vi "e.gate HighSpeedPort Diagnostics Full.vi"(0 "e.gate Configuration":T1 {"StartTime" format="%#.10f"; "dActTimeToSecondFactor" format="%#.10f"; "StartTimeToDayFactor" format="%#_10f"}, 11 "error in (no error)":errorcluster) -> (4 "e.gate Configuration out":T1 {"StartTime" format="%#.10f"; "dActTimeToSecondFactor" format="%#.10f"; "StartTimeToDayFactor" format="%#_10f"}, 6 "e.gate Interface Diagnostic Data":T9={"Interface Kind"=["Fieldbus", "Internal System", "Internal System", "ExternalUART", "ExternalUART", "ExternalUART"], "Interface Index"=[0, 0, 0, 0, 1, 2], "Cycles Count"=[280401, 280401, 280401, 280401, 14024, 280401], "Error Count"=[0, 0, 0, 0, 0, 0], "DeltaTimeS"=[1402.004973, 1402.004982, 1402.004982, 1402.004982, 1402.004983, 1402.004983]}, 8 "e.gate Transport Diagnostic Data":T8, 10 "e.gate Variable Diagnostic Data":T7, 15 "error out":errorcluster)   [LabVIEW 2016]
uses:
  e.gate Diagnostic Interface Data.ctl
  e.gate Diagnostic Transport Data.ctl
  e.gate Diagnostic Variable Data.ctl
  e.gate Configuration.ctl
  e.gate Channel Data.ctl
  e.gate Data Type.ctl
  e.gate Protocol Type.ctl
  e.gate Module  Data.ctl
  e.gateHSP_DLLhandle.ctl
panel:
  out "Remaining Data":u8[](array[numeric])
  out "Structure ID":i8
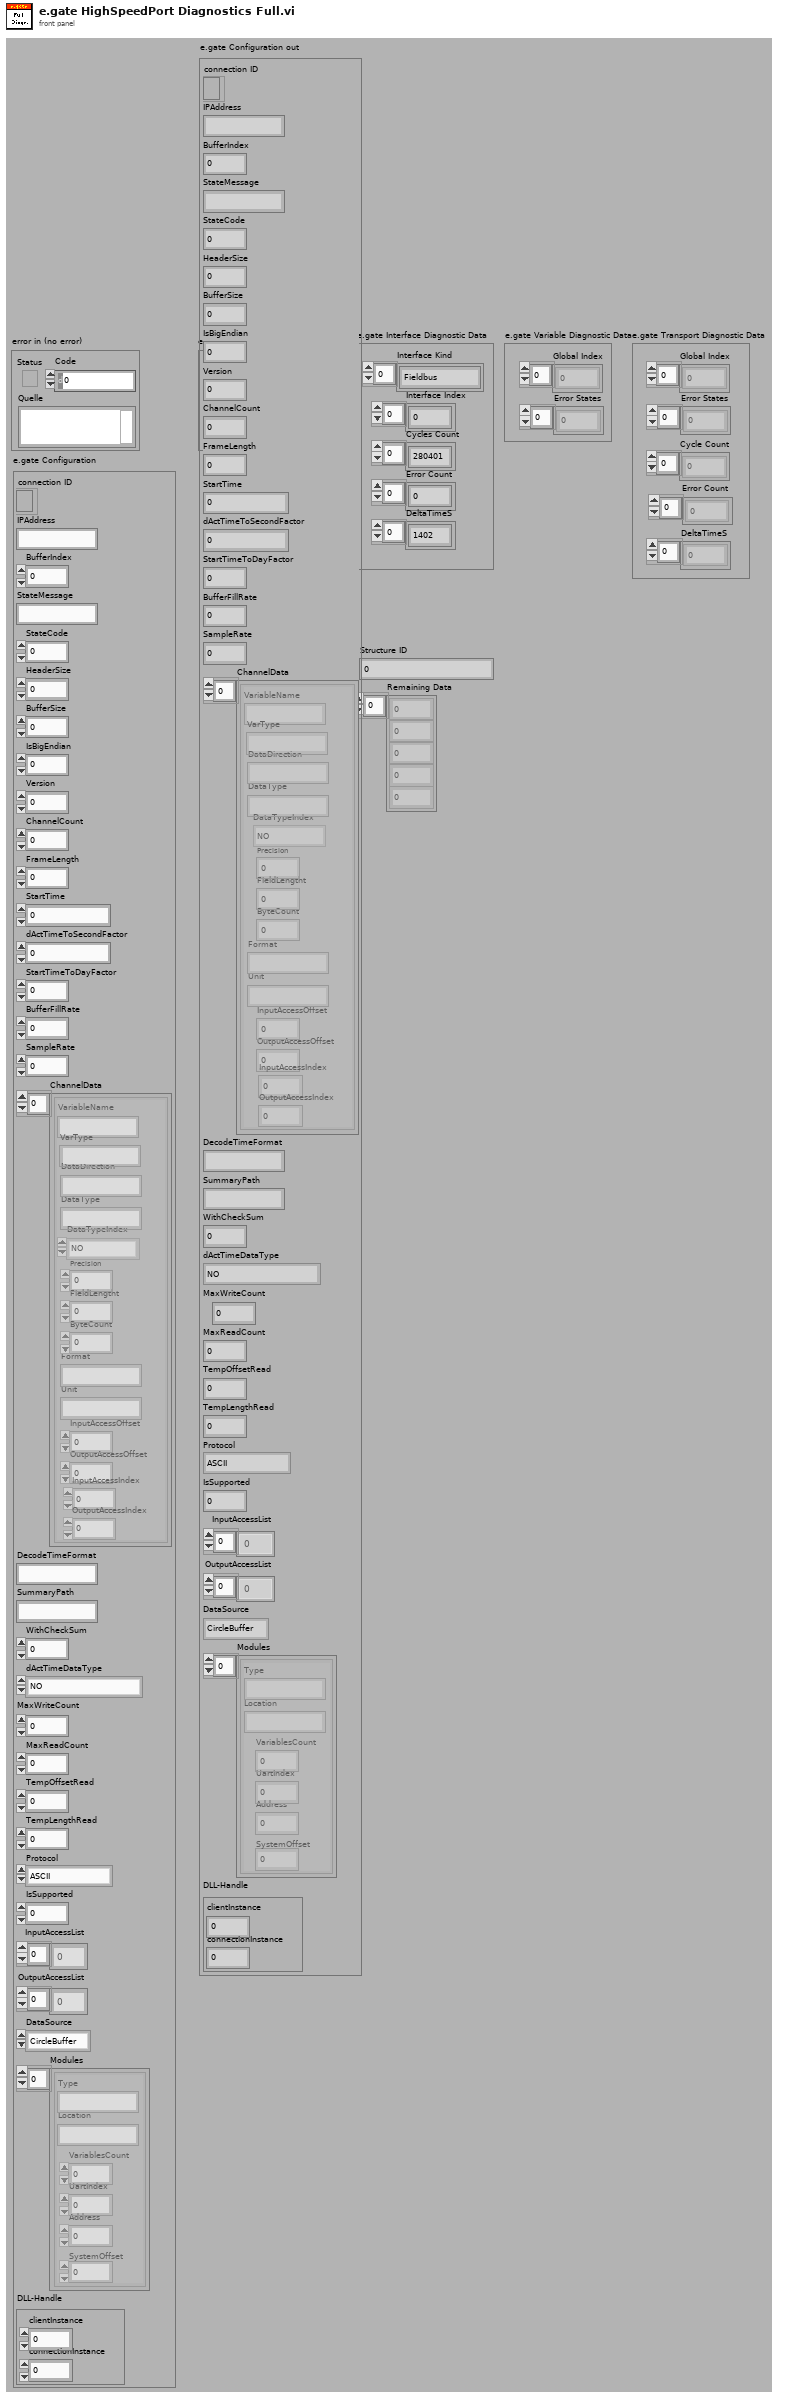
[diagram p1: front panel]
types:
  T1 = typedef "e.gate Configuration.ctl" = cluster{"connection ID":refnum<k5>, "IPAddress":string, "BufferIndex":i32, "StateMessage":string, "StateCode":i8, "HeaderSize":i32, "BufferSize":i32, "IsBigEndian":i32, "Version":i32, "ChannelCount":i32, "FrameLength":i32, "StartTime":dbl, "dActTimeToSecondFactor":dbl, "StartTimeToDayFactor":dbl, "BufferFillRate":dbl, "SampleRate":dbl, "ChannelData":T2[], "DecodeTimeFormat":string, "SummaryPath":string, "WithCheckSum":i32, "dActTimeDataType":T3, "MaxWriteCount":i32, "MaxReadCount":i32, "TempOffsetRead":i32, "TempLengthRead":i32, "Protocol":T4, "IsSupported":i32, "InputAccessList":i32[], "OutputAccessList":i32[], "DataSource":enum16{"CircleBuffer", "test.con Logger", "test.con Archive"}, "Modules":T5[], "DLL-Handle":T6}
  T2 = typedef "e.gate Channel Data.ctl" = cluster{"VariableName":string, "DataDirection":string, "DataType":string, "DataTypeIndex":T3, "Precision":i16, "FieldLengtht":i16, "ByteCount":i32, "Format":string, "Unit":string, "InputAccessOffset":i32, "OutputAccessOffset":i16, "InputAccessIndex":i16, "OutputAccessIndex":i16, "VarType":string}
  T3 = typedef "e.gate Data Type.ctl" = enum16{"NO", "BOOL", "SINT8", "USINT8", "SINT16", "USINT16", "SINT32", "USINT32", "FLOAT", "SET8", "SET16", "SET32", "DOUBLE", "SINT64", "USINT64", "SET64"}
  T4 = typedef "e.gate Protocol Type.ctl" = enum16{"ASCII", "HighspeedPort Online", "HighspeedPort Buffer", "eGateHighspeedPortDLL "}
  T5 = typedef "e.gate Module  Data.ctl" = cluster{"Type":string, "Location":string, "VariablesCount":i16, "UartIndex":i16, "Address":i16, "SystemOffset":i16}
  T6 = typedef "e.gateHSP_DLLhandle.ctl" = cluster{"clientInstance":i32, "connectionInstance":i32}
  T7 = typedef "e.gate Diagnostic Variable Data.ctl" = cluster{"Global Index":i16[], "Error States":i16[]}
  T8 = typedef "e.gate Diagnostic Transport Data.ctl" = cluster{"Global Index":i16[], "Error States":i16[], "Cycle Count":i32[], "Error Count":i32[], "DeltaTimeS":dbl[]}
  T9 = typedef "e.gate Diagnostic Interface Data.ctl" = cluster{"Interface Kind":string[], "Interface Index":i16[], "Cycles Count":i32[], "Error Count":i32[], "DeltaTimeS":dbl[]}
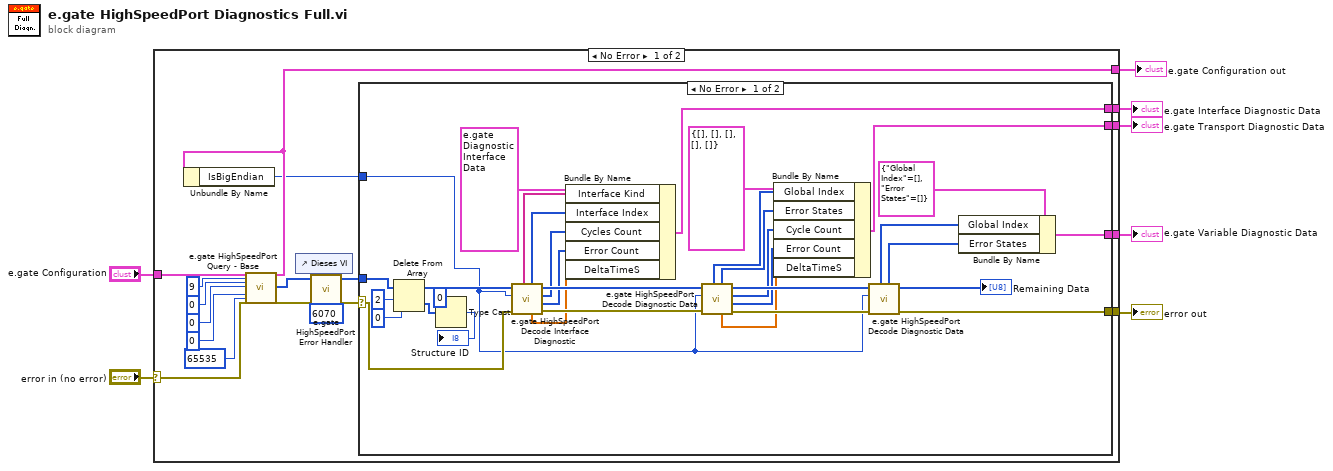
[diagram p0: block diagram]
diagram:
  n1 = case shown="No Error" "error in (no error)" {
    selector: "error in (no error)" -> [w21 w61]
    tunnel: "e.gate Configuration" -> [w26 w62]
    tunnel: [w9 w62] -> w4
    tunnel: [w19 w61] -> w3
    tunnel: [w18 _] -> w7
    tunnel: [w17 _] -> w6
    tunnel: [w16 _] -> w5
    frame No Error {
      n2 = call "e.gate HighSpeedPort Query - Base.vi"("e.gate Configuration in"=w26, "Command"=9, "OffsetWrite"=0, "LengthWrite"=0, "OffsetRead"=0, "LengthRead"=65535, "error in (no error)"=w21) -> ("e.gate Configuration out"=w9:T1, "Data (out binary)"=w13:u8[], "error out"=w12:errorcluster)  [unwired: 3 in, 15 out]
      n3 = Unbundle By Name(w9) -> ("IsBigEndian"=w8:i32)
      n4 = control-ref of="Dieses VI"() -> (w15:refnum<vi>)
      n5 = call "e.gate HighSpeedPort Error Handler.vi"("error code start index"=6070, "VI reference"=w15, "error in (no error)"=w12, "binary data in"=w13) -> ("error out"=w10:errorcluster, "binary out"=w11:u8[])  [unwired: 6 out]
      n6 = case shown="No Error" w10 {
        selector: w10 -> [w28 w60]
        tunnel: [w59 w60] -> w19
        tunnel: [w58 _] -> w18
        tunnel: [w57 _] -> w17
        tunnel: [w56 _] -> w16
        tunnel: w11 -> [w55 _]
        tunnel: w8 -> [w27 _]
        frame No Error {
          n7 = Delete From Array(array=w55, length=2 ("Länge"), index=0 ("Index")) -> (deleted portion=w52:u8[], array with subset deleted=w49:u8[])
          n8 = Type Cast(type=i16 0, x=w52) -> (*(type *) &x=→"Structure ID":i16)
          n9 = call "e.gate HighSpeedPort Decode Interface Diagnostic.vi"("error in"=w28, "IsBigEndian"=w27, "Binary Data in"=w49) -> ("error out"=w47:errorcluster, "Error Count"=w41:i32[], "Cycles Count"=w40:i32[], "Remaining Binary Data"=w48:u8[], "DeltaTimeS"=w42:dbl[], "Interface Index"=w39:i16[], "Interface Kind"=w38:string[])  [unwired: 2 out]
          n10 = Bundle By Name(cluster=T9 {"Interface Kind"=["Fieldbus", "Internal System", "Internal System", "ExternalUART", "ExternalUART", "ExternalUART"], "Interface Index"=[0, 0, 0, 0, 1, 2], "Cycles Count"=[280401, 280401, 280401, 280401, 14024, 280401], "Error Count"=[0, 0, 0, 0, 0, 0], "DeltaTimeS"=[1402.004973, 1402.004982, 1402.004982, 1402.004982, 1402.004983, 1402.004983]} ("e.gate Interface Diagnostic Data"), "Interface Kind"=w38, "Interface Index"=w39, "Cycles Count"=w40, "Error Count"=w41, "DeltaTimeS"=w42) -> (w58:T9)
          n11 = call "e.gate HighSpeedPort Decode Diagnostic Data.vi"("error in"=w47, "IsBigEndian"=w27, "Binary Data in"=w48) -> ("error out"=w45:errorcluster, "Error Count"=w35:i32[], "Cycle Count"=w34:i32[], "Remaining Binary Data"=w46:u8[], "DeltaTimeS"=w36:dbl[], "Error States"=w33:i16[], "Global Indexs"=w32:i16[])  [unwired: 2 out]
          n12 = Bundle By Name(cluster=T8 {"Global Index"=[], "Error States"=[], "Cycle Count"=[], "Error Count"=[], "DeltaTimeS"=[]} ("e.gate Transport Diagnostic Data"), "Global Index"=w32, "Error States"=w33, "Cycle Count"=w34, "Error Count"=w35, "DeltaTimeS"=w36) -> (w57:T8)
          n13 = call "e.gate HighSpeedPort Decode Diagnostic Data.vi"("error in"=w45, "IsBigEndian"=w27, "Binary Data in"=w46) -> ("error out"=w59:errorcluster, "Remaining Binary Data"=→"Remaining Data":u8[], "Error States"=w30:i16[], "Global Indexs"=w29:i16[])  [unwired: 5 out]
          n14 = Bundle By Name(cluster=T7 {"Global Index"=[], "Error States"=[]} ("e.gate Variable Diagnostic Data"), "Global Index"=w29, "Error States"=w30) -> (w56:T7)
        }
        frame Error {
        }
      }
    }
    frame Error {
    }
  }
  "error out" <- w3
  "e.gate Interface Diagnostic Data" <- w7
  "e.gate Transport Diagnostic Data" <- w6
  "e.gate Variable Diagnostic Data" <- w5
  "e.gate Configuration out" <- w4
